vi "KListbox Test.vi"() -> ()   [LabVIEW 2020]
uses:
  KListbox/KListbox.xctl
panel:
  out "Event":string
  in  "stop":bool
  in  "KListbox":cluster{"Row":i32, "Items":string[]}(xcontrol)
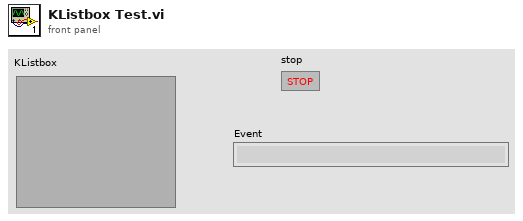
[diagram p1: front panel]
types:
  T1 = typedef "KListbox.xctl/Events.ctl" = cluster{"Items Changed":refnum<user-event>, "List Changed":refnum<user-event>}
  T2 = typedef "KListbox.xctl/Event Action.ctl" = enum16{"Select", "Add", "Delete", "Edit"}
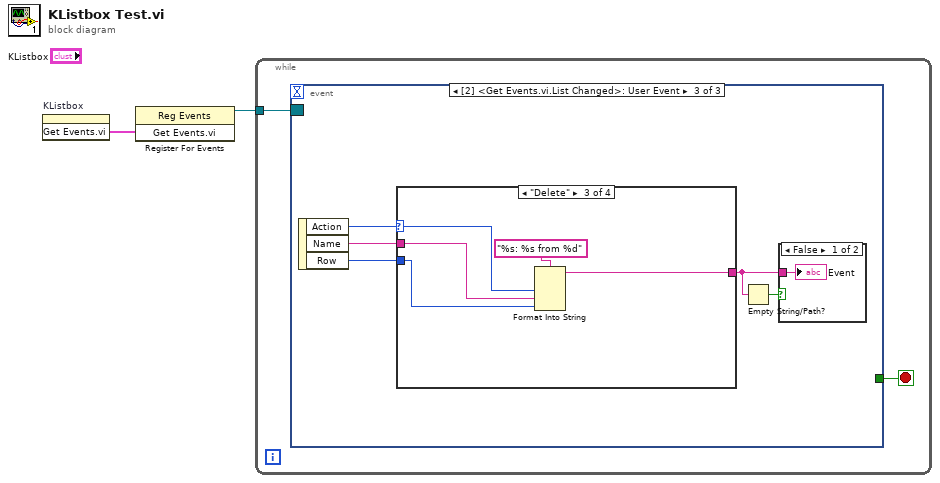
[diagram p0: block diagram]
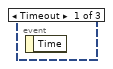
[diagram p2: hidden frame]
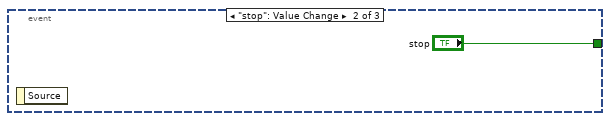
[diagram p3: hidden frame]
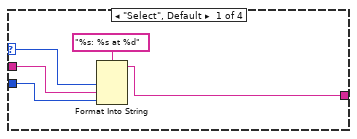
[diagram p5: hidden frame]
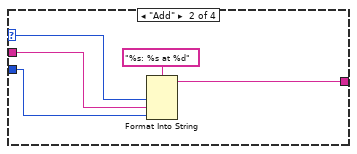
[diagram p6: hidden frame]
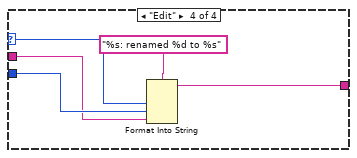
[diagram p7: hidden frame]
diagram:
  n1 = invoke on="KListbox" class="KListbox (strict)" method="Get Events.vi"() -> ("Get Events.vi"=w2:T1)  [unwired: 3 in, 2 out]
  n2 = register-events(w2) -> (reference out=w1:refnum<event-registration>)  [unwired: 2 in, 1 out]
  n3 = while {
    tunnel: w1 -> [w3]
    stop <- w4 stop-if-true
    n4 = event shown="[2] <Get Events.vi.List Changed>: User Event" {
      selector: w3 -> [_ _ _]
      dyn-events: _ -> [_ _ _]
      timeout: _ -> [_ _ _]
      tunnel: [_ "stop" _] -> w4
      event Timeout {
        n5 = event-data() -> ()  [unwired: 1 in, 1 out]
      }
      event "stop": Value Change {
        n6 = event-data() -> ()  [unwired: 1 in, 1 out]
      }
      event User Event {
        n7 = event-data() -> ("Action"=w10:T2, "Name"=w9:string, "Row"=w8:i32)  [unwired: 1 in]
        n8 = case shown="\"Delete\"" w10 {
          selector: w10 -> [w15 w20 w25 w30]
          tunnel: w9 -> [w14 w19 w22 w27]
          tunnel: w8 -> [w13 w18 w23 w28]
          tunnel: [w12 w17 w24 w29] -> w7
          frame "Select", Default {
            n9 = Format Into String(format string="%s: %s at %d", w15, w14, w13) -> (resulting string=w12:string)  [unwired: 2 in, 1 out]
          }
          frame "Add" {
            n10 = Format Into String(format string="%s: %s at %d", w20, w19, w18) -> (resulting string=w17:string)  [unwired: 2 in, 1 out]
          }
          frame "Delete" {
            n11 = Format Into String(format string="%s: %s from %d", w25, w22, w23) -> (resulting string=w24:string)  [unwired: 2 in, 1 out]
          }
          frame "Edit" {
            n12 = Format Into String(format string="%s: renamed %d to %s", w30, w28, w27) -> (resulting string=w29:string)  [unwired: 2 in, 1 out]
          }
        }
        n13 = Empty String/Path?(string/path=w7) -> (empty?=w6:bool)
        n14 = case shown="False" w6 {
          tunnel: w7 -> [w11 _]
          frame False {
            "Event" <- w11
          }
          frame True {
          }
        }
      }
    }
  }
